vi "RUSHShoot.vi"(1 "In Cluster":T2) -> (0 "Out Cluster":T1)   [LabVIEW 2012]
panel:
  in  "Highest POT pos":dbl=4.2
  in  "Lowest POT pos":dbl=2.1
  in  "ShootPOTToPowConst":dbl=1.0
  in  "Vision Speed Const":dbl=0.75
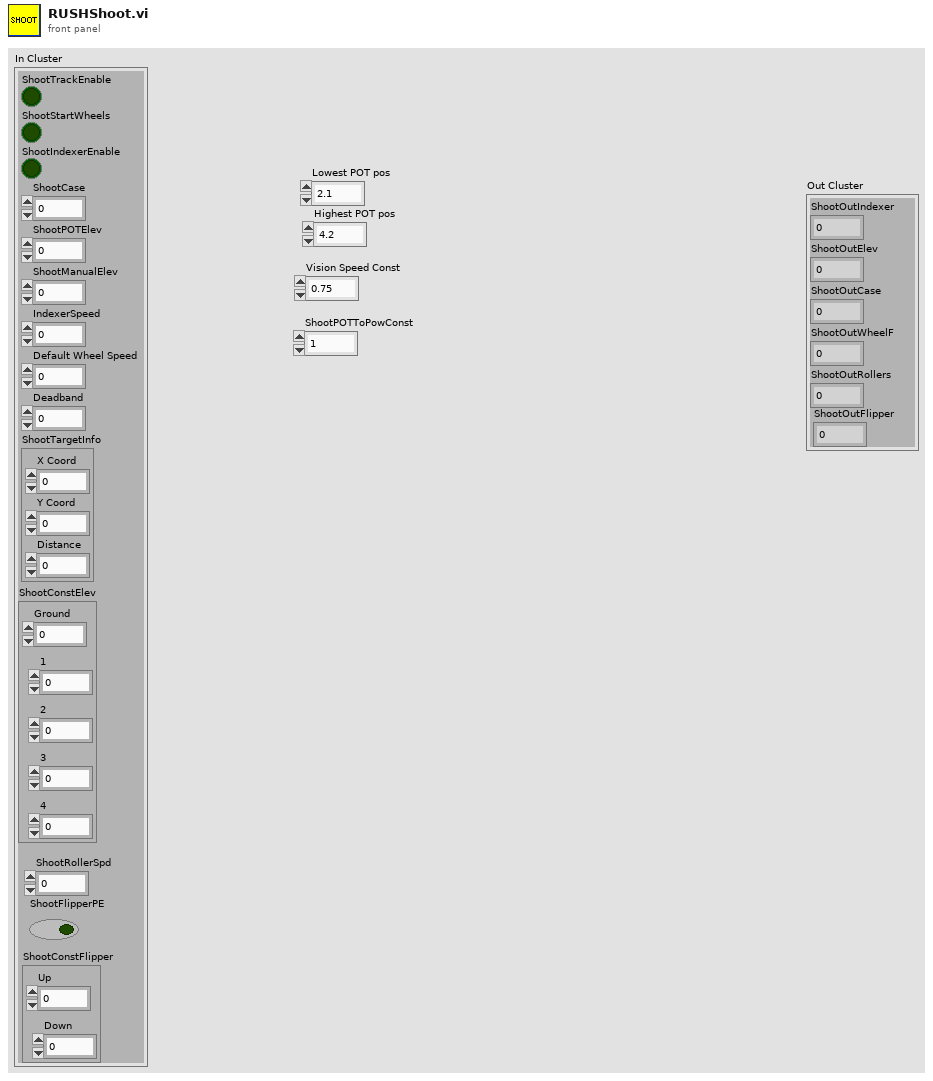
[diagram p1: front panel]
types:
  T1 = cluster{"ShootOutIndexer":dbl, "ShootOutElev":dbl, "ShootOutCase":dbl, "ShootOutWheelF":dbl, "ShootOutRollers":dbl, "ShootOutFlipper":dbl}
  T2 = cluster{"ShootTrackEnable":bool, "ShootStartWheels":bool, "ShootIndexerEnable":bool, "ShootCase":dbl, "ShootPOTElev":dbl, "ShootManualElev":dbl, "IndexerSpeed":dbl, "Default Wheel Speed":dbl, "Deadband":dbl, "ShootTargetInfo":cluster{"X Coord":dbl, "Y Coord":dbl, "Distance":dbl}, "ShootConstElev":cluster{"1":dbl, "2":dbl, "3":dbl, "4":dbl, "Ground":dbl}, "ShootRollerSpd":dbl, "ShootFlipperPE":bool, "ShootConstFlipper":cluster{"Down":dbl, "Up":dbl}}
  T3 = cluster{"X Coord":dbl, "Y Coord":dbl, "Distance":dbl}
  T4 = cluster{"1":dbl, "2":dbl, "3":dbl, "4":dbl, "Ground":dbl}
  T5 = cluster{"f":dbl, "y":dbl, "f":dbl, "f":dbl, "f":dbl, "Down":dbl}
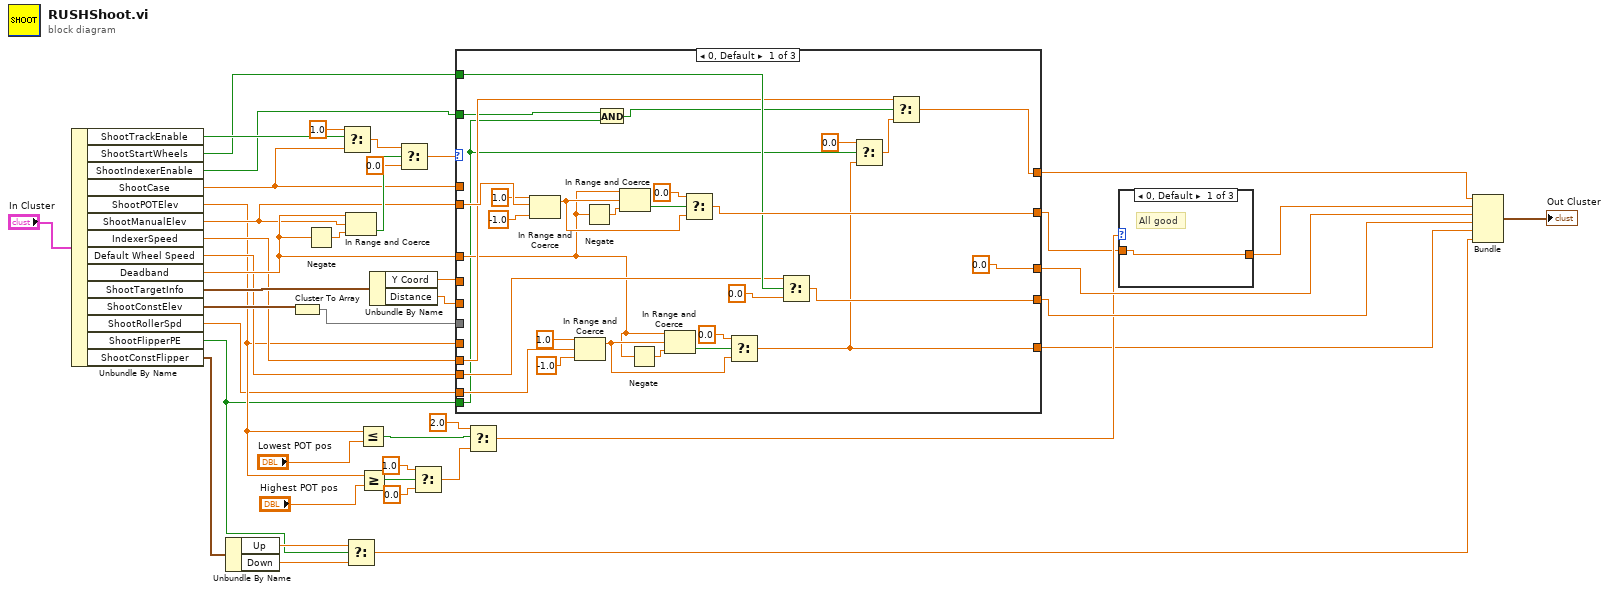
[diagram p0: block diagram]
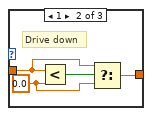
[diagram p2: hidden frame]
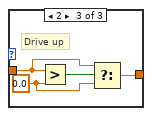
[diagram p3: hidden frame]
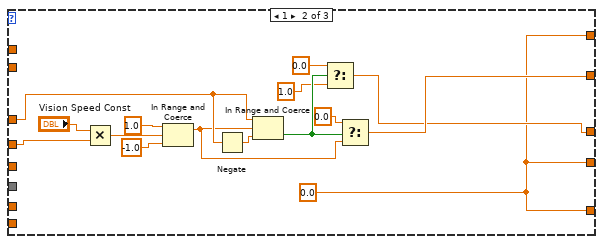
[diagram p4: hidden frame]
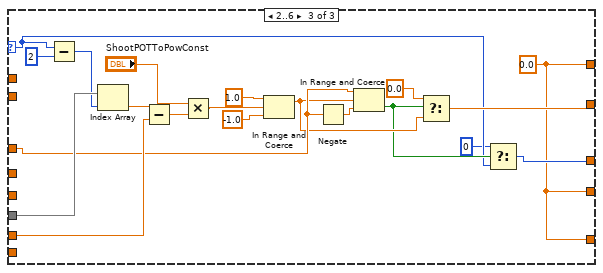
[diagram p5: hidden frame]
diagram:
  n1 = Unbundle By Name("In Cluster") -> ("ShootTrackEnable"=w42:bool, "ShootStartWheels"=w30:bool, "ShootIndexerEnable"=w29:bool, "ShootCase"=w31:dbl, "ShootPOTElev"=w18:dbl, "ShootManualElev"=w28:dbl, "IndexerSpeed"=w21:dbl, "Default Wheel Speed"=w20:dbl, "Deadband"=w32:dbl, "ShootTargetInfo"=w35:T3, "ShootConstElev"=w27:T4, "ShootRollerSpd"=w7:dbl, "ShootFlipperPE"=w1:bool, "ShootConstFlipper"=w4:cluster{"Down":dbl, "Up":dbl})
  n2 = Unbundle By Name(w4) -> ("Up"=w3:dbl, "Down"=w5:dbl)
  n3 = Cluster To Array(cluster=w27) -> (array=w26:dbl[])
  n4 = Negate(x=w32) -> (-x=w39:dbl)
  n5 = Select(t=1.0, s=w42, f=w31) -> (s? t:f=w40:dbl)
  n6 = In Range and Coerce(upper limit=w32, x=w28, lower limit=w39) -> (In Range?=w38:bool)  [unwired: 1 out]
  n7 = Select(t=w3, s=w1, f=w5) -> (s? t:f=w2:dbl)
  n8 = Less Or Equal?(x=w18, y="Lowest POT pos") -> (x <= y?=w12:bool)
  n9 = Greater Or Equal?(x=w18, y="Highest POT pos") -> (x >= y?=w16:bool)
  n10 = Unbundle By Name(w35) -> ("Y Coord"=w34:dbl, "Distance"=w33:dbl)
  n11 = Select(t=w40, s=w38, f=0.0) -> (s? t:f=w36:dbl)
  n12 = Select(t=1.0, s=w16, f=0.0) -> (s? t:f=w13:dbl)
  n13 = case shown="0, Default" w36 {
    selector: w36 -> [_ _ w91]
    tunnel: w34 -> [_ w86 _]
    tunnel: w33 -> [_ _ _]
    tunnel: w32 -> [w50 w81 w96]
    tunnel: [0.0 ("upper limit") w75 w89] -> w24
    tunnel: w31 -> [_ _ _]
    tunnel: [w65 w76 w93] -> w9
    tunnel: [w62 w73 w88] -> w23
    tunnel: [w72 w73 w88] -> w25
    tunnel: w30 -> [w63 _ _]
    tunnel: w29 -> [w49 _ _]
    tunnel: w28 -> [w69 _ _]
    tunnel: w26 -> [_ _ w106]
    tunnel: w18 -> [_ _ w103]
    tunnel: w21 -> [w58 _ _]
    tunnel: w20 -> [w59 _ _]
    tunnel: w7 -> [w51 _ _]
    tunnel: [w45 w73 w88] -> w6
    tunnel: w1 -> [w47 _ _]
    frame 0, Default {
      n14 = In Range and Coerce(upper limit=1.0, x=w69, lower limit=-1.0 ("upper limit")) -> (coerced(x)=w66:dbl)  [unwired: 1 out]
      n15 = In Range and Coerce(upper limit=1.0, x=w51, lower limit=-1.0 ("upper limit")) -> (coerced(x)=w56:dbl)  [unwired: 1 out]
      n16 = Negate(x=w50) -> (-x=w70:dbl)
      n17 = And(x=w49, y=w47) -> (x .and. y?=w48:bool)
      n18 = In Range and Coerce(upper limit=w50, x=w66, lower limit=w70) -> (In Range?=w68:bool)  [unwired: 1 out]
      n19 = Negate(x=w50) -> (-x=w53:dbl)
      n20 = In Range and Coerce(upper limit=w50, x=w56, lower limit=w53) -> (In Range?=w54:bool)  [unwired: 1 out]
      n21 = Select(t=0.0, s=w68, f=w66) -> (s? t:f=w65:dbl)
      n22 = Select(t=0.0, s=w54, f=w56) -> (s? t:f=w45:dbl)
      n23 = Select(t=w59, s=w63, f=0.0 ("t")) -> (s? t:f=w62:dbl)
      n24 = Select(t=0.0, s=w47, f=w45) -> (s? t:f=w44:dbl)
      n25 = Select(t=w58, s=w48, f=w44) -> (s? t:f=w72:dbl)
    }
    frame 1 {
      w73 = 0.0
      n26 = Multiply(x="Vision Speed Const", y=w86) -> (x*y=w85:dbl)
      n27 = In Range and Coerce(upper limit=1.0, x=w85, lower limit=-1.0 ("upper limit")) -> (coerced(x)=w79:dbl)  [unwired: 1 out]
      n28 = Negate(x=w81) -> (-x=w82:dbl)
      n29 = In Range and Coerce(upper limit=w81, x=w79, lower limit=w82) -> (In Range?=w78:bool)  [unwired: 1 out]
      n30 = Select(t=0.0, s=w78, f=1.0) -> (s? t:f=w75:dbl)
      n31 = Select(t=0.0, s=w78, f=w79) -> (s? t:f=w76:dbl)
    }
    frame 2..6 {
      w88 = 0.0 ("f")
      n32 = Subtract(x=w91, y=2) -> (x-y=w105:i32)
      n33 = Index Array(array=w106, index=w105) -> (element=w104:dbl)
      n34 = Subtract(x=w104, y=w103) -> (x-y=w102:dbl)
      n35 = Multiply(x="ShootPOTToPowConst", y=w102) -> (x*y=w97:dbl)
      n36 = In Range and Coerce(upper limit=1.0, x=w97, lower limit=-1.0 ("upper limit")) -> (coerced(x)=w94:dbl)  [unwired: 1 out]
      n37 = Negate(x=w96) -> (-x=w98:dbl)
      n38 = In Range and Coerce(upper limit=w96, x=w94, lower limit=w98) -> (In Range?=w92:bool)  [unwired: 1 out]
      n39 = Select(t=0.0, s=w92, f=w94) -> (s? t:f=w93:dbl)
      n40 = Select(t=0, s=w92, f=w91) -> (s? t:f=w89:i32)
    }
  }
  n41 = Select(t=2.0, s=w12, f=w13) -> (s? t:f=w10:dbl)
  n42 = case shown="0, Default" w10 {
    tunnel: w9 -> [w108 w110 w114]
    tunnel: [w108 w109 w113] -> w8
    frame 0, Default {
      # "All good"
    }
    frame 1 {
      w111 = 0.0 ("y")
      # "Drive down"
      n43 = Less?(x=w110, y=w111) -> (x < y?=w112:bool)
      n44 = Select(t=w110, s=w112, f=w111) -> (s? t:f=w109:dbl)
    }
    frame 2 {
      w115 = 0.0 ("y")
      # "Drive up"
      n45 = Greater?(x=w114, y=w115) -> (0:w116:bool)
      n46 = Select(t=w114, s=w116, f=w115) -> (s? t:f=w113:dbl)
    }
  }
  n47 = Bundle("f"=w25, "y"=w8, "f"=w24, "f"=w23, "f"=w6, "Down"=w2) -> (→"Out Cluster":T5)  [unwired: 1 in]
